vi "audio-discrimination-task.vi"() -> ()   [LabVIEW 2015]
uses:
  states-enum.ctl
  <vilib>/Utility/file.llb/Read Delimited Spreadsheet (I64).vi
panel:
  out "s? t:f":T1
  out "element":i64
  out "Trials":string
  out "Reward (mL)":string
  out "Licks":string
  out "CR":string
  out "Acc":string
  out "Miss":string
  out "FA":string
  out "Hits":string
  out "Current State":string
  out "Time Elapsed":dbl format="%<%H:%M:%S>t"
  in  "Tab Control":enum32{"Required", "Optional"}(tab)
  in  "Max Time (s)":dbl
  in  "Number of trials":string(combo)
  in  "Max number of \nconsecutive trials":string(combo)
  in  "Data Saving Directory":path
  in  "Animal Name":string
  in  "Sequence Directory":path
  in  "Assay Description":string
  in  "Recording Location":string
  in  "Trial delay (ms)":dbl
  in  "Punish Time (s)":dbl
  in  "Trial window (ms)":dbl
  in  "ITI lower (s)":dbl
  in  "ITI upper (s)":dbl
  out "trials":i64[](array[numeric])
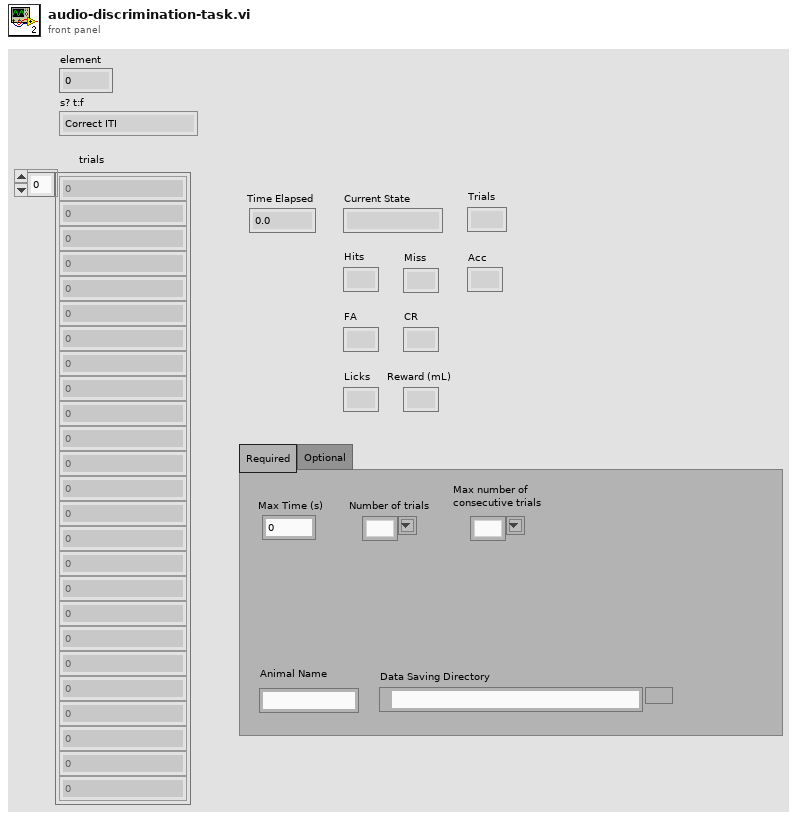
[diagram p1: front panel]
types:
  T1 = typedef "states-enum.ctl" = enum16{"Correct ITI", "Incorrect ITI", "Trial 0", "Trial 1", "Stop", ""}
  T2 = cluster{"ITI upper (s)":dbl, "ITI lower (s)":dbl, "Punish Time (s)":dbl, "Trial window (ms)":dbl, "Trial delay (ms)":dbl, "Max Time (s)":dbl}
  T3 = cluster{"appended path":path, "relative seconds":dbl, "Current Trial Index":i32, "Accuracy":i32, "Hits":i32, "Miss":i32, "False Alarm":i32, "Correct Rejection":i32, "Licks":i32, "Reward (ml)":i32}
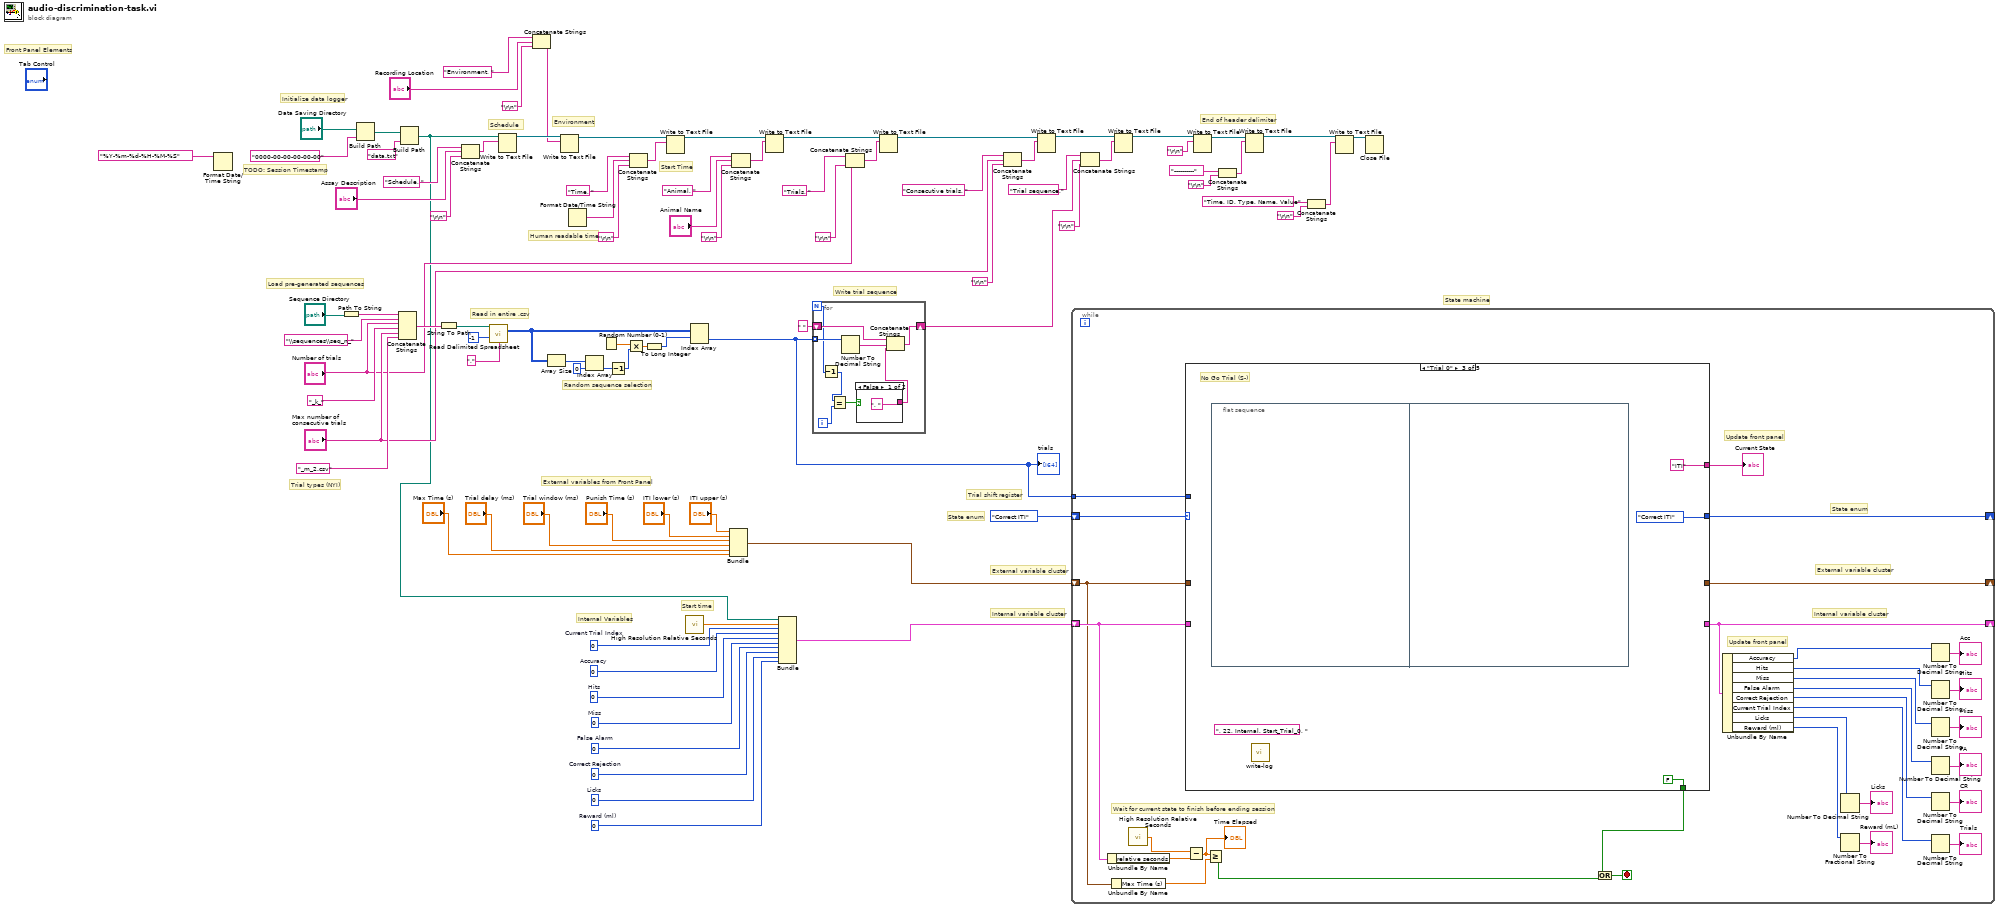
[diagram p0: block diagram]
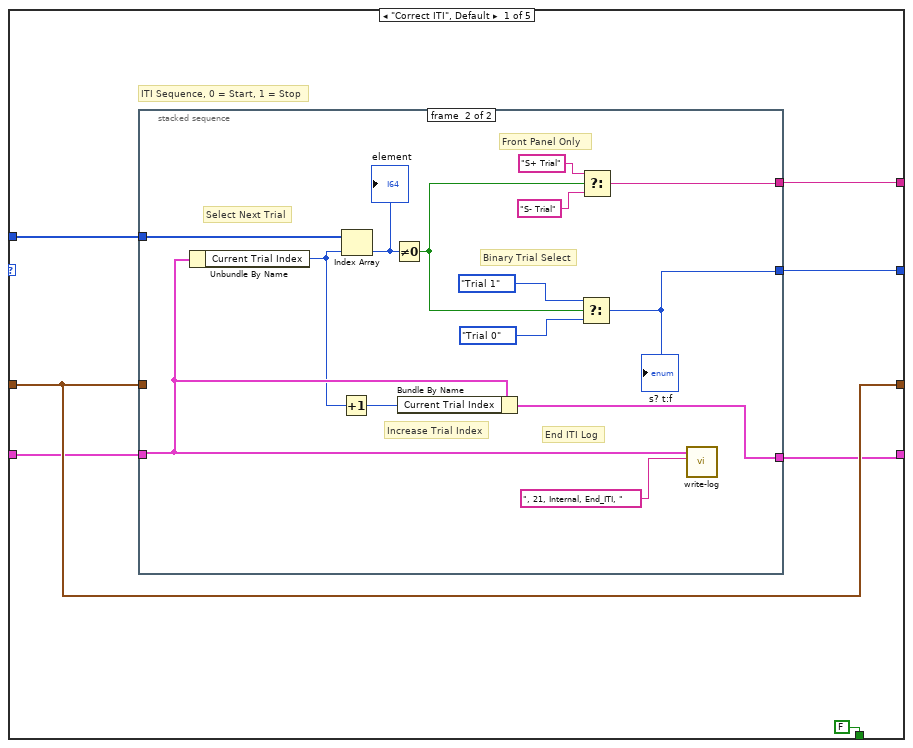
[diagram p2: hidden frame]
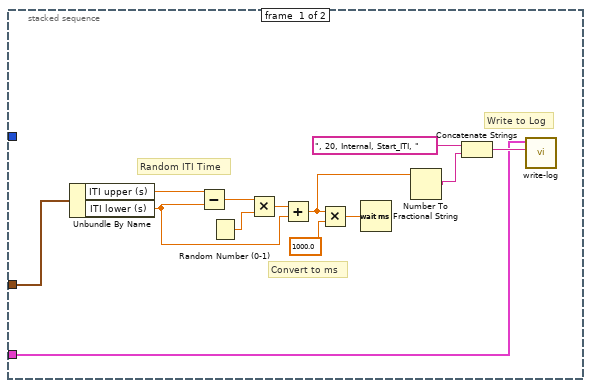
[diagram p3: hidden frame]
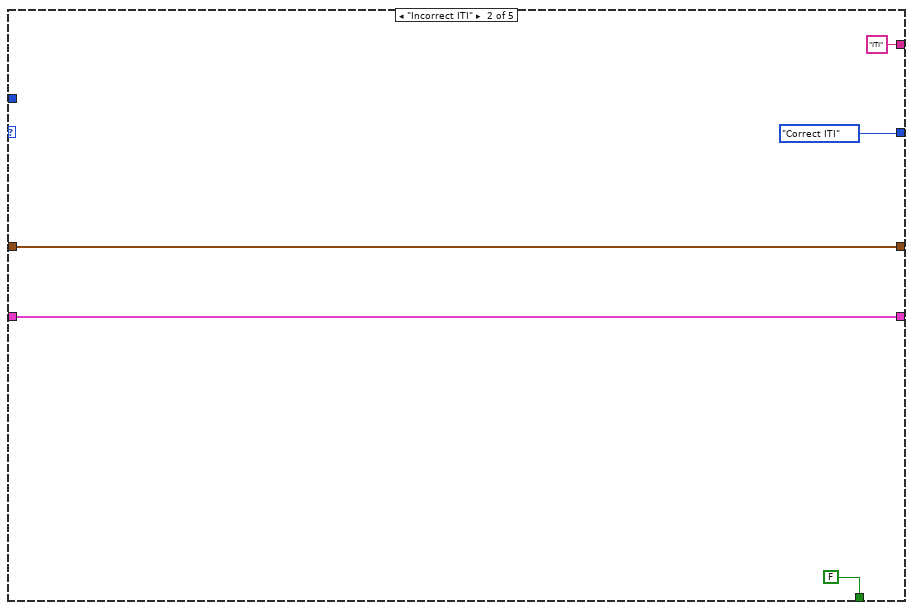
[diagram p4: hidden frame]
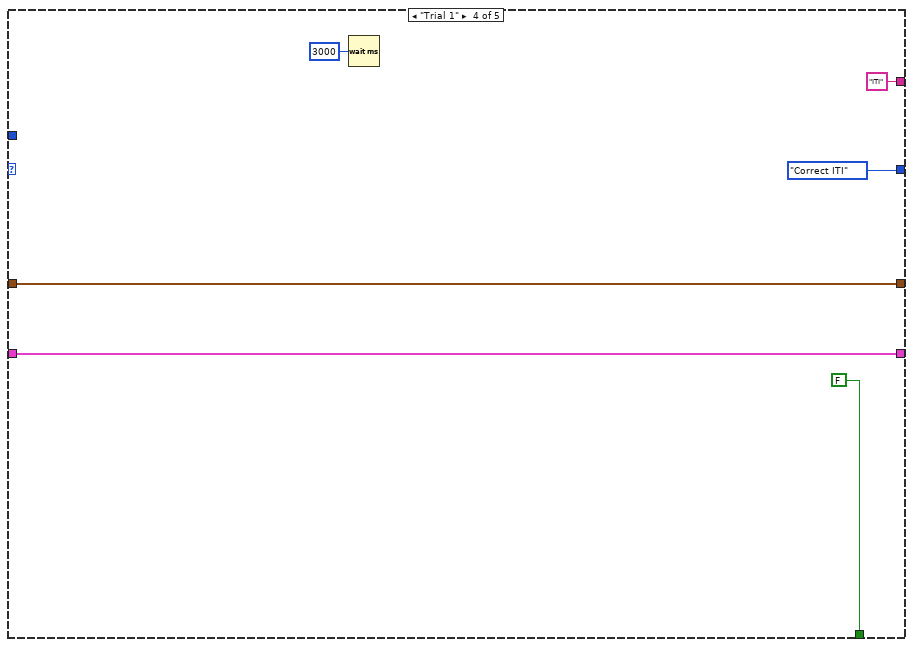
[diagram p5: hidden frame]
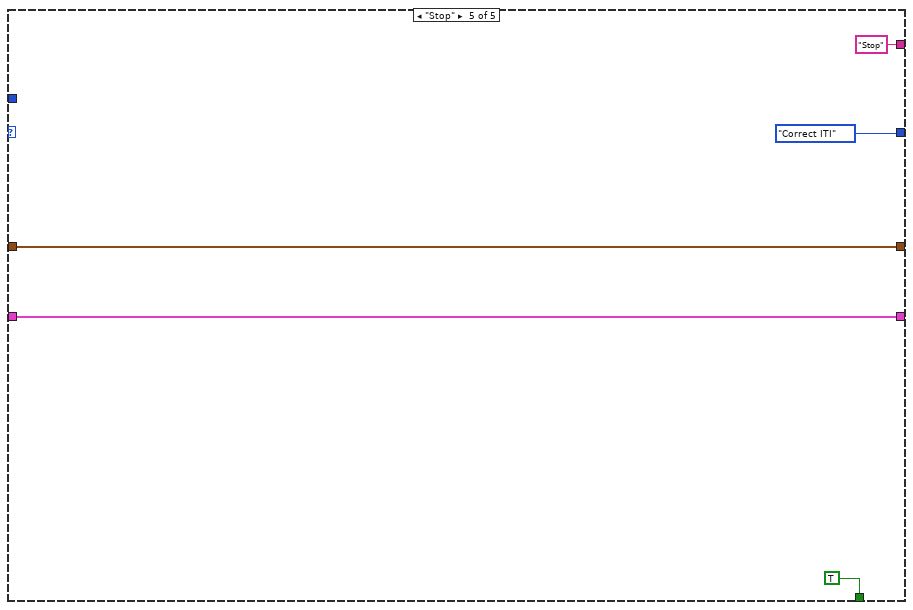
[diagram p6: hidden frame]
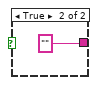
[diagram p7: hidden frame]
diagram:
  w9 = 0  # Reward (ml)
  w10 = 0  # Licks
  w11 = 0  # Correct Rejection
  w12 = 0  # False Alarm
  w15 = 0  # Accuracy
  w13 = 0  # Miss
  w14 = 0  # Hits
  w16 = 0  # Current Trial Index
  # "Start time"
  # "Internal Variables"
  # "External variables from Front Panel"
  # "External variable cluster"
  # "Internal variable cluster"
  # "State enum"
  # "Trial shift register"
  # "State machine"
  # "Front Panel Elements"
  # "Write trial sequence"
  # "Human readable time"
  # "End of header delimiter"
  # "Start Time"
  # "Environment"
  # "Schedule"
  # "Initialize data logger"
  # "TODO: Session Timestamp"
  # "Random sequence selection"
  # "Trial types (NYI)"
  # "Read in entire .csv"
  # "Load pre-generated sequences"
  n1 = Format Date/Time String(time format string (%c)="%Y-%m-%d-%H-%M-%S") -> ()  [unwired: 2 in, 1 out]
  n2 = Path To String(path="Sequence Directory") -> (string=w83:string)
  n3 = Build Path(base path="Data Saving Directory", name or relative path="0000-00-00-00-00-00") -> (appended path=w71:path)
  n4 = Concatenate Strings(w83, "\\sequences\\seq_n_", "Number of trials", "_k_" ("string"), "Max number of \nconsecutive trials", "_m_2.csv" ("string")) -> (w79:string)
  n5 = Build Path(base path=w71, name or relative path="data.txt") -> (appended path=w6:path)
  n6 = String To Path(string=w79) -> (path=w80:path)
  n7 = Concatenate Strings("Schedule, " ("string"), "Assay Description", "\r\n") -> (w67:string)
  n8 = call-poly <vilib>:"Read Delimited Spreadsheet.vi"("file path (dialog if empty)"=w80, "number of rows (all:-1)"=-1, "delimiter (\\t)"="," ("delimiter (\\t)")) -> ("all rows"=w74:i64[][])  [unwired: 7 in, 5 out]
  n9 = Write to Text File(file (use dialog)=w6, text=w67) -> (refnum out=w69:refnum<file>)  [unwired: 2 in, 2 out]
  n10 = Concatenate Strings("Environment, " ("string"), "Recording Location", "\r\n") -> (w63:string)
  n11 = Array Size(array=w74) -> (size(s)=w78:i32[])
  n12 = Write to Text File(file (use dialog)=w69, text=w63) -> (refnum out=w61:refnum<file>)  [unwired: 2 in, 2 out]
  n13 = Format Date/Time String() -> (date/time string=w36:string)  [unwired: 3 in]
  n14 = Index Array(array=w78, index=0) -> (element=w76:i32)
  n15 = Random Number (0-1)() -> (number: 0 to 1=w86:dbl)
  n16 = Decrement(x=w76) -> (x-1=w75:i32)
  n17 = Multiply(x=w86, y=w75) -> (x*y=w85:dbl)
  n18 = Concatenate Strings("Time, " ("string"), w36, "\r\n") -> (w58:string)
  n19 = To Long Integer(number=w85) -> (32bit integer=w73:i32)
  n20 = Write to Text File(file (use dialog)=w61, text=w58) -> (refnum out=w57:refnum<file>)  [unwired: 2 in, 2 out]
  n21 = call <vilib>:"High Resolution Relative Seconds.vi"() -> ("relative seconds"=w18:dbl)
  n22 = Index Array(array=w74, index (row)=w73) -> (element=w8:i64[])  [unwired: 1 in]
  "trials" <- w8
  n23 = Bundle("ITI upper (s)"="ITI upper (s)", "ITI lower (s)"="ITI lower (s)", "Punish Time (s)"="Punish Time (s)", "Trial window (ms)"="Trial window (ms)", "Trial delay (ms)"="Trial delay (ms)", "Max Time (s)"="Max Time (s)") -> (w19:T2)  [unwired: 1 in]
  n24 = Concatenate Strings("Animal, " ("string"), "Animal Name", "\r\n") -> (w54:string)
  n25 = Write to Text File(file (use dialog)=w57, text=w54) -> (refnum out=w46:refnum<file>)  [unwired: 2 in, 2 out]
  n26 = Bundle("appended path"=w6, "relative seconds"=w18, "Current Trial Index"=w16, "Accuracy"=w15, "Hits"=w14, "Miss"=w13, "False Alarm"=w12, "Correct Rejection"=w11, "Licks"=w10, "Reward (ml)"=w9) -> (w17:T3)  [unwired: 1 in]
  n27 = for {
    N -> [w90]
    shift-right: [w94] -> w29
    shift-left: " " -> [w95]
    tunnel: w8 -> [w97] mode=indexing
    i -> [w93]
    n28 = Decrement(x=w90) -> (x-1=w89:i32)
    n29 = Equal?(x=w89, y=w93) -> (x = y?=w92:bool)
    n30 = Number To Decimal String(number=w97) -> (decimal integer string=w96:string)  [unwired: 1 in]
    n31 = case shown="False" w92 {
      tunnel: [", " ("string") "" ("string")] -> w91
      frame False {
      }
      frame True {
      }
    }
    n32 = Concatenate Strings(w95, w96, w91) -> (w94:string)
  }
  n33 = Concatenate Strings("Trials, " ("string"), "Number of trials", "\r\n") -> (w50:string)
  n34 = Write to Text File(file (use dialog)=w46, text=w50) -> (refnum out=w45:refnum<file>)  [unwired: 2 in, 2 out]
  n35 = Concatenate Strings("Consecutive trials, " ("string"), "Max number of \nconsecutive trials", "\r\n") -> (w47:string)
  n36 = Write to Text File(file (use dialog)=w45, text=w47) -> (refnum out=w34:refnum<file>)  [unwired: 2 in, 2 out]
  n37 = while {
    shift-right: [w129] -> _
    shift-left: states-enum."Correct ITI" -> [w130]
    shift-right: [w128] -> _
    shift-left: w19 -> [w117]
    shift-right: [w116] -> _
    shift-left: w17 -> [w127]
    tunnel: w8 -> [w119]
    stop <- w123 stop-if-true
    # "State enum"
    # "Internal variable cluster"
    # "External variable cluster"
    # "Update front panel"
    # "Update front panel"
    # "Wait for current state to finish before ending session"
    n38 = Unbundle By Name(w127) -> ("relative seconds"=w125:dbl)
    n39 = Unbundle By Name(w117) -> ("Max Time (s)"=w124:dbl)
    n40 = call <vilib>:"High Resolution Relative Seconds.vi"() -> ("relative seconds"=w126:dbl)
    n41 = case shown="\"Trial 0\"" w130 {
      tunnel: [FALSE FALSE FALSE FALSE TRUE] -> w122
      tunnel: [w132 states-enum."Correct ITI" states-enum."Correct ITI" states-enum."Correct ITI" states-enum."Correct ITI"] -> w129
      tunnel: w119 -> [w135 _ _ _ _]
      tunnel: w117 -> [w136 w168 _ w176 w182]
      tunnel: [w136 w168 _ w176 w182] -> w128
      tunnel: w127 -> [w134 w169 _ w175 w181]
      tunnel: [w133 w169 _ w175 w181] -> w116
      tunnel: [w131 "ITI" "ITI" "ITI" "Stop"] -> w118
      frame "Correct ITI", Default {
        # "ITI Sequence, 0 = Start, 1 = Stop"
        n42 = stacked-sequence {
          tunnel: w136 -> [w138 _]
          tunnel: w134 -> [w139 w162]
          tunnel: w135 -> [_ w163]
          tunnel: [_ w159] -> w133
          tunnel: [_ w155] -> w132
          tunnel: [_ w151] -> w131
          frame #0 {
            # "Write to Log"
            # "Convert to ms"
            # "Random ITI Time"
            n43 = Unbundle By Name(w138) -> ("ITI upper (s)"=w140:dbl, "ITI lower (s)"=w144:dbl)
            n44 = Subtract(x=w140, y=w144) -> (x-y=w141:dbl)
            n45 = Random Number (0-1)() -> (number: 0 to 1=w142:dbl)
            n46 = Multiply(x=w141, y=w142) -> (x*y=w143:dbl)
            n47 = Add(x=w143, y=w144) -> (x+y=w149:dbl)
            n48 = Multiply(x=w149, y=1000.0) -> (x*y=w146:dbl)
            n49 = Wait (ms)(milliseconds to wait=w146) -> ()  [unwired: 1 out]
            n50 = Number To Fractional String(number=w149) -> (F-format string=w150:string)  [unwired: 3 in]
            n51 = Concatenate Strings(", 20, Internal, Start_ITI, " ("text"), w150) -> (w148:string)
            n52 = call "write-log.vi"("Write Text"=w148, "Internal Cluster"=w139) -> ()  [unwired: 10 in]
          }
          frame #1 {
            # "Binary Trial Select"
            # "Front Panel Only"
            # "Increase Trial Index"
            # "Select Next Trial"
            # "End ITI Log"
            n53 = Unbundle By Name(w162) -> ("Current Trial Index"=w160:i32)
            n54 = Increment(x=w160) -> (x+1=w161:i32)
            n55 = Index Array(array=w163, index=w160) -> (element=w158:i64)
            "element" <- w158
            n56 = Not Equal To 0?(x=w158) -> (x != 0?=w154:bool)
            n57 = Bundle By Name(cluster=w162, "Current Trial Index"=w161) -> (w159:T3)
            n58 = Select(t=states-enum."Trial 1", s=w154, f=states-enum."Trial 0") -> (s? t:f=w155:T1)
            "s? t:f" <- w155
            n59 = Select(t="S+ Trial", s=w154, f="S- Trial") -> (s? t:f=w151:string)
            n60 = call "write-log.vi"("Write Text"=", 21, Internal, End_ITI, " ("text"), "Internal Cluster"=w162) -> ()  [unwired: 10 in]
          }
        }
      }
      frame "Incorrect ITI" {
      }
      frame "Trial 0" {
        (unwired) ", 22, Internal, Start_Trial_0, " ("text")
        # "No Go Trial (S-)"
        n61 = flat-sequence {
          frame #0 {
          }
          frame #1 {
          }
        }
        n62 = call "write-log.vi"() -> ()  [unwired: 12 in]
      }
      frame "Trial 1" {
        n63 = Wait (ms)(milliseconds to wait=u32 3000) -> ()  [unwired: 1 out]
      }
      frame "Stop" {
      }
    }
    "Current State" <- w118
    n64 = Subtract(x=w126, y=w125) -> (x-y=w120:dbl)
    "Time Elapsed" <- w120
    n65 = Greater Or Equal?(x=w120, y=w124) -> (x >= y?=w121:bool)
    n66 = Or(x=w122, y=w121) -> (x .or. y?=w123:bool)
    n67 = Unbundle By Name(w116) -> ("Accuracy"=w100:i32, "Hits"=w101:i32, "Miss"=w102:i32, "False Alarm"=w103:i32, "Correct Rejection"=w104:i32, "Current Trial Index"=w105:i32, "Licks"=w106:i32, "Reward (ml)"=w107:i32)
    n68 = Number To Decimal String(number=w106) -> (decimal integer string=→"Licks":string)  [unwired: 1 in]
    n69 = Number To Fractional String(number=w107) -> (F-format string=→"Reward (mL)":string)  [unwired: 3 in]
    n70 = Number To Decimal String(number=w100) -> (decimal integer string=→"Acc":string)  [unwired: 1 in]
    n71 = Number To Decimal String(number=w101) -> (decimal integer string=→"Hits":string)  [unwired: 1 in]
    n72 = Number To Decimal String(number=w102) -> (decimal integer string=→"Miss":string)  [unwired: 1 in]
    n73 = Number To Decimal String(number=w103) -> (decimal integer string=→"FA":string)  [unwired: 1 in]
    n74 = Number To Decimal String(number=w104) -> (decimal integer string=→"CR":string)  [unwired: 1 in]
    n75 = Number To Decimal String(number=w105) -> (decimal integer string=→"Trials":string)  [unwired: 1 in]
  }
  n76 = Concatenate Strings("Trial sequence," ("string"), w29, "\r\n") -> (w32:string)
  n77 = Write to Text File(file (use dialog)=w34, text=w32) -> (refnum out=w33:refnum<file>)  [unwired: 2 in, 2 out]
  n78 = Write to Text File(file (use dialog)=w33, text="\r\n") -> (refnum out=w40:refnum<file>)  [unwired: 2 in, 2 out]
  n79 = Concatenate Strings("----------" ("string"), "\r\n") -> (w39:string)
  n80 = Write to Text File(file (use dialog)=w40, text=w39) -> (refnum out=w3:refnum<file>)  [unwired: 2 in, 2 out]
  n81 = Concatenate Strings("Time, ID, Type, Name, Value" ("string"), "\r\n") -> (w1:string)
  n82 = Write to Text File(file (use dialog)=w3, text=w1) -> (refnum out=w2:refnum<file>)  [unwired: 2 in, 2 out]
  n83 = Close File(refnum=w2) -> ()  [unwired: 1 in, 2 out]
